vi "CTRE_CANifier_ConfigGetSlot.vi"(6 "timeoutMs":i32=50, 8 "error in (no error)":errorcluster, 11 "CANifierDevRef":T3) -> (0 "error out":errorcluster, 2 "CANifier Configuration":T1={"velocityMeasurementPeriod"=100, "velocityMeasurementWindow"=0, "clearPositionOnLimitF"=FALSE, "clearPositionOnLimitR"=FALSE, "clearPositionOnLimitQuadIdx"=FALSE, "CustomParam"={"customParam 0"=0, "customParam 1"=0}} {"velocityMeasurementPeriod" items=["Period_1Ms"=1, "Period_2Ms"=2, "Period_5Ms"=5, "Period_10Ms"=10, "Period_20Ms"=20, "Period_25Ms"=25, "Period_50Ms"=50, "Period_100Ms"=100]}, 3 "CANifierDevRef":T3)   [LabVIEW 2017]
doc: "Gets all persistant settings"
uses:
  <vilib>/Rock Robotics/WPI/ThirdParty/Phoenix-LabVIEW/CANifier/CTRE_CANifier_DeviceRef.ctl
  <vilib>/Rock Robotics/WPI/ThirdParty/Phoenix-LabVIEW/CANifier/CTRE_CANifier_Configurables.ctl
  <vilib>/Rock Robotics/WPI/ThirdParty/Phoenix-LabVIEW/Controls/CTRE_Phoenix_CustomParamConfiguration.ctl
  <vilib>/Rock Robotics/WPI/ThirdParty/Phoenix-LabVIEW/Controls/CTRE_Phoenix_Params.ctl
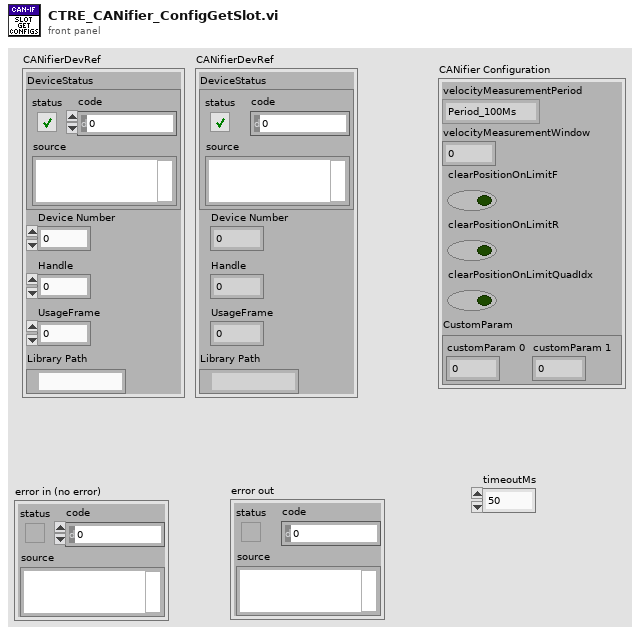
[diagram p1: front panel]
types:
  T1 = typedef "CTRE_CANifier_Configurables.ctl" = cluster{"velocityMeasurementPeriod":u16, "velocityMeasurementWindow":i32, "clearPositionOnLimitF":bool, "clearPositionOnLimitR":bool, "clearPositionOnLimitQuadIdx":bool, "CustomParam":T2}
  T2 = typedef "CTRE_Phoenix_CustomParamConfiguration.ctl" = cluster{"customParam 0":i32, "customParam 1":i32}
  T3 = typedef "CTRE_CANifier_DeviceRef.ctl" = cluster{"DeviceStatus":errorcluster, "Device Number":u8, "Handle":u64, "UsageFrame":u32, "Library Path":path}
  T4 = typedef "CTRE_Phoenix_Params.ctl" = u16
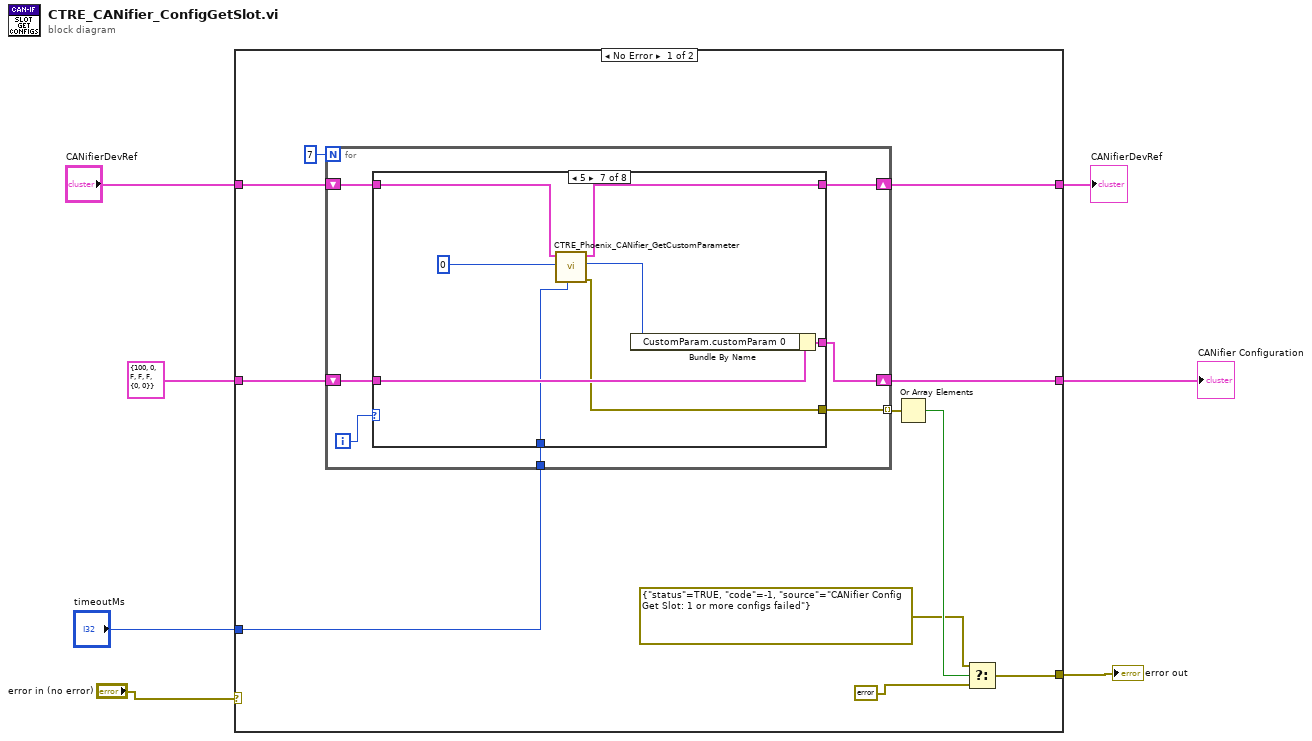
[diagram p0: block diagram]
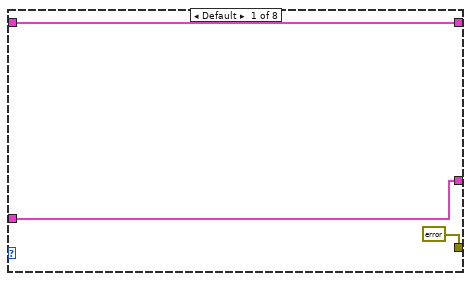
[diagram p2: hidden frame]
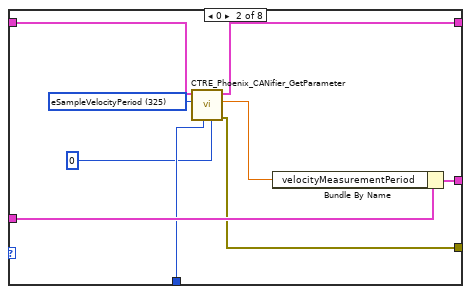
[diagram p3: hidden frame]
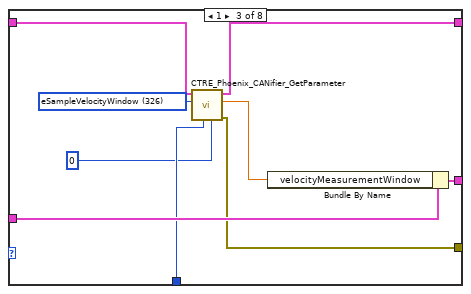
[diagram p4: hidden frame]
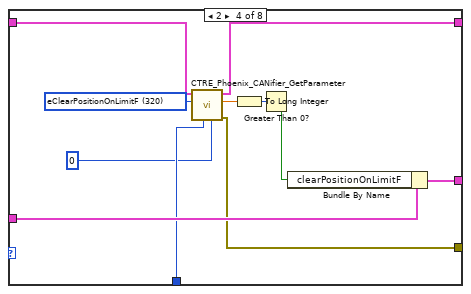
[diagram p5: hidden frame]
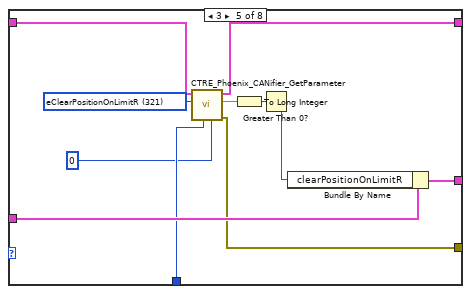
[diagram p6: hidden frame]
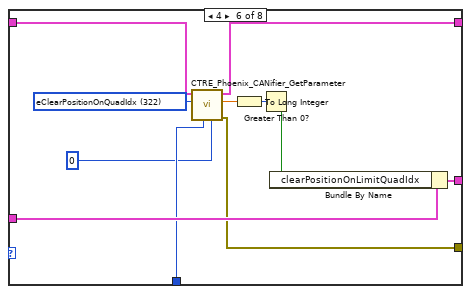
[diagram p7: hidden frame]
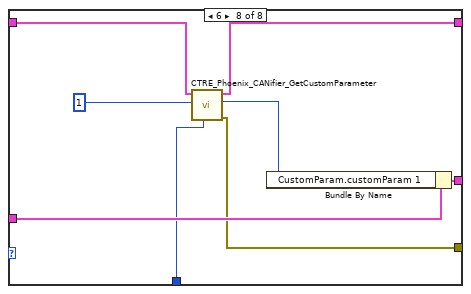
[diagram p8: hidden frame]
diagram:
  n1 = case shown="No Error" "error in (no error)" {
    selector: "error in (no error)" -> [_ w98]
    tunnel: T1 {"velocityMeasurementPeriod"=100, "velocityMeasurementWindow"=0, "clearPositionOnLimitF"=FALSE, "clearPositionOnLimitR"=FALSE, "clearPositionOnLimitQuadIdx"=FALSE, "CustomParam"={"customParam 0"=0, "customParam 1"=0}} ("CANifier Configuration 2") -> [w16 w96]
    tunnel: "CANifierDevRef" -> [w18 w97]
    tunnel: [w17 w97] -> w5
    tunnel: "timeoutMs" -> [w15 _]
    tunnel: [w12 w98] -> w3
    tunnel: [w8 w96] -> w2
    frame No Error {
      n2 = for {
        N: 7 -> [_]
        shift-right: [w22] -> w17
        shift-left: w18 -> [w23]
        tunnel: w15 -> [w21]
        tunnel: [w20] -> w13 mode=indexing
        shift-right: [w19] -> w8
        shift-left: w16 -> [w24]
        i -> [w25]
        n3 = case shown="5" w25 {
          tunnel: w24 -> [w26 w37 w46 w57 w68 w79 w87 w95]
          tunnel: w23 -> [w28 w36 w45 w56 w67 w78 w86 w94]
          tunnel: [w28 w35 w44 w55 w66 w77 w85 w93] -> w22
          tunnel: w21 -> [_ w32 w41 w53 w64 w75 w84 w92]
          tunnel: [errorcluster {"status"=FALSE, "code"=0, "source"=""} ("error out") w30 w39 w51 w62 w73 w82 w90] -> w20
          tunnel: [w26 w29 w38 w50 w61 w72 w81 w89] -> w19
          frame Default {
          }
          frame 0 {
            w34 = T4 325 items=["eOnBoot_BrakeMode"=31, "eQuadFilterEn"=91, "eQuadIdxPolarity"=108, "eClearPositionOnIdx"=100, "eMotionProfileHasUnderrunErr"=119, "eMotionProfileTrajectoryPointDurationMs"=120, "eClearPosOnLimitF"=144, "eClearPosOnLimitR"=145, "eStatusFramePeriod"=300, "eOpenLoopRamp"=301, "eClosedLoopRamp"=302, "eNeutralDeadband"=303, "ePeakPosOutput"=305, "eNominalPosOutput"=306, "ePeakNegOutput"=307, "eNominalNegOutput"=308, "eProfileParamSlot_P"=310, "eProfileParamSlot_I"=311, "eProfileParamSlot_D"=312, "eProfileParamSlot_F"=313, "eProfileParamSlot_IZone"=314, "eProfileParamSlot_AllowableErr"=315, "eProfileParamSlot_MaxIAccum"=316, "eProfileParamSlot_PeakOutput"=317, "eClearPositionOnLimitF"=320, "eClearPositionOnLimitR"=321, "eClearPositionOnQuadIdx"=322, "eSampleVelocityPeriod"=325, "eSampleVelocityWindow"=326, "eFeedbackSensorType"=330, "eSelectedSensorPosition"=331, "eFeedbackNotContinuous"=332, "eRemoteSensorSource"=333, "eRemoteSensorDeviceID"=334, "eSensorTerm"=335, "eRemoteSensorClosedLoopDisableNeutralOnLOS"=336, "ePIDLoopPolarity"=337, "ePIDLoopPeriod"=338, "eSelectedSensorCoefficient"=339, "eForwardSoftLimitThreshold"=340, "eReverseSoftLimitThreshold"=341, "eForwardSoftLimitEnable"=342, "eReverseSoftLimitEnable"=343, "eNominalBatteryVoltage"=350, "eBatterVoltageFilterSize"=351, "eContinuousCurrentLimitAmps"=360, "eContinuousCurrentLimitMs"=361, "ePeakCurrentLimitAmps"=362, "eClosedLoopIAccum"=370, "eCustomParam"=380, "eStickyFaults"=390, "eAnalogPosition"=400, "eQuadraturePosition"=401, "ePulseWidthPosition"=402, "eMotMag_Accel"=410, "eMotMag_VelCruise"=411, "eLimitSwitchSource"=421, "eLimitSwitchNormClosedAndDis"=422, "eLimitSwitchDisabledNeutralOnLOS"=423, "eLimitSwitchRemoteDevID"=424, "eSoftLimitDisabledNeutralOnLOS"=425, "ePulseWidthPeriod_EdgesPerRot"=430, "ePulseWidthPeriod_FilterWindowSz"=431] ("Parameter")
            n4 = call <vilib>:"CTRE_Phoenix_CANifier_GetParameter.vi"("ordinal"=0, "timeoutMs"=w32, "Parameter"=w34, "CTRE_CANifier_DeviceRef"=w36) -> ("error out"=w30:errorcluster, "value"=w33:dbl, "CTRE_CANifier_DeviceRef"=w35:T3)  [unwired: 5 in]
            n5 = Bundle By Name(cluster=w37, "velocityMeasurementPeriod"=w33) -> (w29:T1)
          }
          frame 1 {
            w43 = T4 326 items=["eOnBoot_BrakeMode"=31, "eQuadFilterEn"=91, "eQuadIdxPolarity"=108, "eClearPositionOnIdx"=100, "eMotionProfileHasUnderrunErr"=119, "eMotionProfileTrajectoryPointDurationMs"=120, "eClearPosOnLimitF"=144, "eClearPosOnLimitR"=145, "eStatusFramePeriod"=300, "eOpenLoopRamp"=301, "eClosedLoopRamp"=302, "eNeutralDeadband"=303, "ePeakPosOutput"=305, "eNominalPosOutput"=306, "ePeakNegOutput"=307, "eNominalNegOutput"=308, "eProfileParamSlot_P"=310, "eProfileParamSlot_I"=311, "eProfileParamSlot_D"=312, "eProfileParamSlot_F"=313, "eProfileParamSlot_IZone"=314, "eProfileParamSlot_AllowableErr"=315, "eProfileParamSlot_MaxIAccum"=316, "eProfileParamSlot_PeakOutput"=317, "eClearPositionOnLimitF"=320, "eClearPositionOnLimitR"=321, "eClearPositionOnQuadIdx"=322, "eSampleVelocityPeriod"=325, "eSampleVelocityWindow"=326, "eFeedbackSensorType"=330, "eSelectedSensorPosition"=331, "eFeedbackNotContinuous"=332, "eRemoteSensorSource"=333, "eRemoteSensorDeviceID"=334, "eSensorTerm"=335, "eRemoteSensorClosedLoopDisableNeutralOnLOS"=336, "ePIDLoopPolarity"=337, "ePIDLoopPeriod"=338, "eSelectedSensorCoefficient"=339, "eForwardSoftLimitThreshold"=340, "eReverseSoftLimitThreshold"=341, "eForwardSoftLimitEnable"=342, "eReverseSoftLimitEnable"=343, "eNominalBatteryVoltage"=350, "eBatterVoltageFilterSize"=351, "eContinuousCurrentLimitAmps"=360, "eContinuousCurrentLimitMs"=361, "ePeakCurrentLimitAmps"=362, "eClosedLoopIAccum"=370, "eCustomParam"=380, "eStickyFaults"=390, "eAnalogPosition"=400, "eQuadraturePosition"=401, "ePulseWidthPosition"=402, "eMotMag_Accel"=410, "eMotMag_VelCruise"=411, "eLimitSwitchSource"=421, "eLimitSwitchNormClosedAndDis"=422, "eLimitSwitchDisabledNeutralOnLOS"=423, "eLimitSwitchRemoteDevID"=424, "eSoftLimitDisabledNeutralOnLOS"=425, "ePulseWidthPeriod_EdgesPerRot"=430, "ePulseWidthPeriod_FilterWindowSz"=431] ("Parameter")
            n6 = call <vilib>:"CTRE_Phoenix_CANifier_GetParameter.vi"("ordinal"=0, "timeoutMs"=w41, "Parameter"=w43, "CTRE_CANifier_DeviceRef"=w45) -> ("error out"=w39:errorcluster, "value"=w42:dbl, "CTRE_CANifier_DeviceRef"=w44:T3)  [unwired: 5 in]
            n7 = Bundle By Name(cluster=w46, "velocityMeasurementWindow"=w42) -> (w38:T1)
          }
          frame 2 {
            w54 = T4 320 items=["eOnBoot_BrakeMode"=31, "eQuadFilterEn"=91, "eQuadIdxPolarity"=108, "eClearPositionOnIdx"=100, "eMotionProfileHasUnderrunErr"=119, "eMotionProfileTrajectoryPointDurationMs"=120, "eClearPosOnLimitF"=144, "eClearPosOnLimitR"=145, "eStatusFramePeriod"=300, "eOpenLoopRamp"=301, "eClosedLoopRamp"=302, "eNeutralDeadband"=303, "ePeakPosOutput"=305, "eNominalPosOutput"=306, "ePeakNegOutput"=307, "eNominalNegOutput"=308, "eProfileParamSlot_P"=310, "eProfileParamSlot_I"=311, "eProfileParamSlot_D"=312, "eProfileParamSlot_F"=313, "eProfileParamSlot_IZone"=314, "eProfileParamSlot_AllowableErr"=315, "eProfileParamSlot_MaxIAccum"=316, "eProfileParamSlot_PeakOutput"=317, "eClearPositionOnLimitF"=320, "eClearPositionOnLimitR"=321, "eClearPositionOnQuadIdx"=322, "eSampleVelocityPeriod"=325, "eSampleVelocityWindow"=326, "eFeedbackSensorType"=330, "eSelectedSensorPosition"=331, "eFeedbackNotContinuous"=332, "eRemoteSensorSource"=333, "eRemoteSensorDeviceID"=334, "eSensorTerm"=335, "eRemoteSensorClosedLoopDisableNeutralOnLOS"=336, "ePIDLoopPolarity"=337, "ePIDLoopPeriod"=338, "eSelectedSensorCoefficient"=339, "eForwardSoftLimitThreshold"=340, "eReverseSoftLimitThreshold"=341, "eForwardSoftLimitEnable"=342, "eReverseSoftLimitEnable"=343, "eNominalBatteryVoltage"=350, "eBatterVoltageFilterSize"=351, "eContinuousCurrentLimitAmps"=360, "eContinuousCurrentLimitMs"=361, "ePeakCurrentLimitAmps"=362, "eClosedLoopIAccum"=370, "eCustomParam"=380, "eStickyFaults"=390, "eAnalogPosition"=400, "eQuadraturePosition"=401, "ePulseWidthPosition"=402, "eMotMag_Accel"=410, "eMotMag_VelCruise"=411, "eLimitSwitchSource"=421, "eLimitSwitchNormClosedAndDis"=422, "eLimitSwitchDisabledNeutralOnLOS"=423, "eLimitSwitchRemoteDevID"=424, "eSoftLimitDisabledNeutralOnLOS"=425, "ePulseWidthPeriod_EdgesPerRot"=430, "ePulseWidthPeriod_FilterWindowSz"=431] ("Parameter")
            n8 = call <vilib>:"CTRE_Phoenix_CANifier_GetParameter.vi"("ordinal"=0, "timeoutMs"=w53, "Parameter"=w54, "CTRE_CANifier_DeviceRef"=w56) -> ("error out"=w51:errorcluster, "value"=w49:dbl, "CTRE_CANifier_DeviceRef"=w55:T3)  [unwired: 5 in]
            n9 = To Long Integer(number=w49) -> (32bit integer=w48:i32)
            n10 = Greater Than 0?(x=w48) -> (x > 0?=w47:bool)
            n11 = Bundle By Name(cluster=w57, "clearPositionOnLimitF"=w47) -> (w50:T1)
          }
          frame 3 {
            w65 = T4 321 items=["eOnBoot_BrakeMode"=31, "eQuadFilterEn"=91, "eQuadIdxPolarity"=108, "eClearPositionOnIdx"=100, "eMotionProfileHasUnderrunErr"=119, "eMotionProfileTrajectoryPointDurationMs"=120, "eClearPosOnLimitF"=144, "eClearPosOnLimitR"=145, "eStatusFramePeriod"=300, "eOpenLoopRamp"=301, "eClosedLoopRamp"=302, "eNeutralDeadband"=303, "ePeakPosOutput"=305, "eNominalPosOutput"=306, "ePeakNegOutput"=307, "eNominalNegOutput"=308, "eProfileParamSlot_P"=310, "eProfileParamSlot_I"=311, "eProfileParamSlot_D"=312, "eProfileParamSlot_F"=313, "eProfileParamSlot_IZone"=314, "eProfileParamSlot_AllowableErr"=315, "eProfileParamSlot_MaxIAccum"=316, "eProfileParamSlot_PeakOutput"=317, "eClearPositionOnLimitF"=320, "eClearPositionOnLimitR"=321, "eClearPositionOnQuadIdx"=322, "eSampleVelocityPeriod"=325, "eSampleVelocityWindow"=326, "eFeedbackSensorType"=330, "eSelectedSensorPosition"=331, "eFeedbackNotContinuous"=332, "eRemoteSensorSource"=333, "eRemoteSensorDeviceID"=334, "eSensorTerm"=335, "eRemoteSensorClosedLoopDisableNeutralOnLOS"=336, "ePIDLoopPolarity"=337, "ePIDLoopPeriod"=338, "eSelectedSensorCoefficient"=339, "eForwardSoftLimitThreshold"=340, "eReverseSoftLimitThreshold"=341, "eForwardSoftLimitEnable"=342, "eReverseSoftLimitEnable"=343, "eNominalBatteryVoltage"=350, "eBatterVoltageFilterSize"=351, "eContinuousCurrentLimitAmps"=360, "eContinuousCurrentLimitMs"=361, "ePeakCurrentLimitAmps"=362, "eClosedLoopIAccum"=370, "eCustomParam"=380, "eStickyFaults"=390, "eAnalogPosition"=400, "eQuadraturePosition"=401, "ePulseWidthPosition"=402, "eMotMag_Accel"=410, "eMotMag_VelCruise"=411, "eLimitSwitchSource"=421, "eLimitSwitchNormClosedAndDis"=422, "eLimitSwitchDisabledNeutralOnLOS"=423, "eLimitSwitchRemoteDevID"=424, "eSoftLimitDisabledNeutralOnLOS"=425, "ePulseWidthPeriod_EdgesPerRot"=430, "ePulseWidthPeriod_FilterWindowSz"=431] ("Parameter")
            n12 = call <vilib>:"CTRE_Phoenix_CANifier_GetParameter.vi"("ordinal"=0, "timeoutMs"=w64, "Parameter"=w65, "CTRE_CANifier_DeviceRef"=w67) -> ("error out"=w62:errorcluster, "value"=w60:dbl, "CTRE_CANifier_DeviceRef"=w66:T3)  [unwired: 5 in]
            n13 = To Long Integer(number=w60) -> (32bit integer=w59:i32)
            n14 = Greater Than 0?(x=w59) -> (x > 0?=w58:bool)
            n15 = Bundle By Name(cluster=w68, "clearPositionOnLimitR"=w58) -> (w61:T1)
          }
          frame 4 {
            w76 = T4 322 items=["eOnBoot_BrakeMode"=31, "eQuadFilterEn"=91, "eQuadIdxPolarity"=108, "eClearPositionOnIdx"=100, "eMotionProfileHasUnderrunErr"=119, "eMotionProfileTrajectoryPointDurationMs"=120, "eClearPosOnLimitF"=144, "eClearPosOnLimitR"=145, "eStatusFramePeriod"=300, "eOpenLoopRamp"=301, "eClosedLoopRamp"=302, "eNeutralDeadband"=303, "ePeakPosOutput"=305, "eNominalPosOutput"=306, "ePeakNegOutput"=307, "eNominalNegOutput"=308, "eProfileParamSlot_P"=310, "eProfileParamSlot_I"=311, "eProfileParamSlot_D"=312, "eProfileParamSlot_F"=313, "eProfileParamSlot_IZone"=314, "eProfileParamSlot_AllowableErr"=315, "eProfileParamSlot_MaxIAccum"=316, "eProfileParamSlot_PeakOutput"=317, "eClearPositionOnLimitF"=320, "eClearPositionOnLimitR"=321, "eClearPositionOnQuadIdx"=322, "eSampleVelocityPeriod"=325, "eSampleVelocityWindow"=326, "eFeedbackSensorType"=330, "eSelectedSensorPosition"=331, "eFeedbackNotContinuous"=332, "eRemoteSensorSource"=333, "eRemoteSensorDeviceID"=334, "eSensorTerm"=335, "eRemoteSensorClosedLoopDisableNeutralOnLOS"=336, "ePIDLoopPolarity"=337, "ePIDLoopPeriod"=338, "eSelectedSensorCoefficient"=339, "eForwardSoftLimitThreshold"=340, "eReverseSoftLimitThreshold"=341, "eForwardSoftLimitEnable"=342, "eReverseSoftLimitEnable"=343, "eNominalBatteryVoltage"=350, "eBatterVoltageFilterSize"=351, "eContinuousCurrentLimitAmps"=360, "eContinuousCurrentLimitMs"=361, "ePeakCurrentLimitAmps"=362, "eClosedLoopIAccum"=370, "eCustomParam"=380, "eStickyFaults"=390, "eAnalogPosition"=400, "eQuadraturePosition"=401, "ePulseWidthPosition"=402, "eMotMag_Accel"=410, "eMotMag_VelCruise"=411, "eLimitSwitchSource"=421, "eLimitSwitchNormClosedAndDis"=422, "eLimitSwitchDisabledNeutralOnLOS"=423, "eLimitSwitchRemoteDevID"=424, "eSoftLimitDisabledNeutralOnLOS"=425, "ePulseWidthPeriod_EdgesPerRot"=430, "ePulseWidthPeriod_FilterWindowSz"=431] ("Parameter")
            n16 = call <vilib>:"CTRE_Phoenix_CANifier_GetParameter.vi"("ordinal"=0, "timeoutMs"=w75, "Parameter"=w76, "CTRE_CANifier_DeviceRef"=w78) -> ("error out"=w73:errorcluster, "value"=w71:dbl, "CTRE_CANifier_DeviceRef"=w77:T3)  [unwired: 5 in]
            n17 = To Long Integer(number=w71) -> (32bit integer=w70:i32)
            n18 = Greater Than 0?(x=w70) -> (x > 0?=w69:bool)
            n19 = Bundle By Name(cluster=w79, "clearPositionOnLimitQuadIdx"=w69) -> (w72:T1)
          }
          frame 5 {
            n20 = call <vilib>:"CTRE_Phoenix_CANifier_GetCustomParameter.vi"("timeoutMs"=w84, "paramIndex"=0 ("ordinal"), "CTRE_CANifier_DeviceRef"=w86) -> ("error out"=w82:errorcluster, "readValue"=w80:i32, "CTRE_CANifier_DeviceRef"=w85:T3)  [unwired: 6 in]
            n21 = Bundle By Name(cluster=w87, "CustomParam.customParam 0"=w80) -> (w81:T1)
          }
          frame 6 {
            n22 = call <vilib>:"CTRE_Phoenix_CANifier_GetCustomParameter.vi"("timeoutMs"=w92, "paramIndex"=1 ("ordinal"), "CTRE_CANifier_DeviceRef"=w94) -> ("error out"=w90:errorcluster, "readValue"=w88:i32, "CTRE_CANifier_DeviceRef"=w93:T3)  [unwired: 6 in]
            n23 = Bundle By Name(cluster=w95, "CustomParam.customParam 1"=w88) -> (w89:T1)
          }
        }
      }
      n24 = Or Array Elements(Boolean array=w13) -> (logical OR=w11:bool)
      n25 = Select(t=errorcluster {"status"=TRUE, "code"=-1, "source"="CANifier Config Get Slot: 1 or more configs failed"} ("error out"), s=w11, f=errorcluster {"status"=FALSE, "code"=0, "source"=""} ("error out")) -> (s? t:f=w12:errorcluster)
    }
    frame Error {
    }
  }
  "CANifierDevRef" <- w5
  "error out" <- w3
  "CANifier Configuration" <- w2
